vi "write_converter_file.vi"(9 "CONVERTER":cluster{dbl, dbl, dbl}, 10 "minutes":dbl, 11 "converter file":path) -> ()   [LabVIEW 2019]
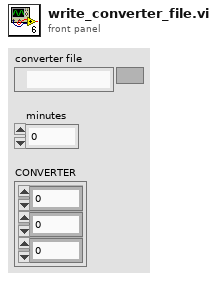
[diagram p1: front panel]
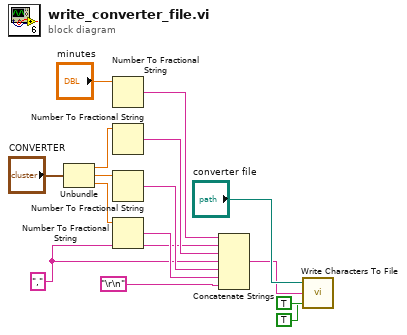
[diagram p0: block diagram]
diagram:
  w2 = "," ("string")
  n1 = Unbundle("CONVERTER") -> (w7:dbl, w8:dbl, w9:dbl)
  n2 = Number To Fractional String(number="minutes") -> (F-format string=w10:string)  [unwired: 3 in]
  n3 = Number To Fractional String(number=w7) -> (F-format string=w11:string)  [unwired: 3 in]
  n4 = Number To Fractional String(number=w8) -> (F-format string=w12:string)  [unwired: 3 in]
  n5 = Number To Fractional String(number=w9) -> (F-format string=w13:string)  [unwired: 3 in]
  n6 = Concatenate Strings(w10, w2, w11, w2, w12, w13, "\r\n") -> (w14:string)
  n7 = call <vilib>:"Write Characters To File.vi"("convert eol? (no:F)"=TRUE, "append to file? (new file:F)"=TRUE, "character string"=w14, "file path (dialog if empty)"="converter file") -> ()  [unwired: 1 in, 1 out]
